vi "SHIFTER - GUI Template.vi"() -> (8 "SHIFTER DATA":T1)   [LabVIEW 2012, in "REx_Springboard.lvlib"]
uses:
  REx_Springboard.lvlib
  TypeDef - SHIFTER - GUI Template.ctl
  Dependencies.llb/Exit Event Ref.ctl
  Dependencies.llb/TLB_Dependencies.lvlib
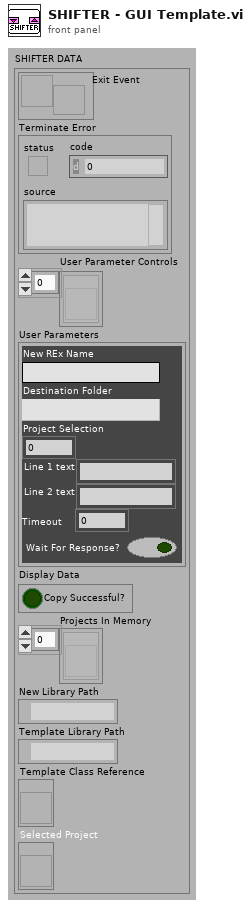
[diagram p1: front panel]
types:
  T1 = typedef "REx_Springboard.lvlib/TypeDef - SHIFTER - GUI Template.ctl" = cluster{"Exit Event":T2, "Terminate Error":errorcluster, "User Parameter Controls":refnum<vi>[], "User Parameters":cluster{"New REx Name":string, "Destination Folder":path, "Project Selection":u16, "Line 1 text":string, "Line 2 text":string, "Timeout":i32, "Wait For Response?":bool}, "Display Data":cluster{"Copy Successful?":bool}, "Projects In Memory":refnum<vi>[], "New Library Path":path, "Template Library Path":path, "Template Class Reference":refnum<vi>, "Selected Project":refnum<vi>}
  T2 = typedef "REx_Springboard.lvlib/TLB_Dependencies.lvlib/Exit Event Ref.ctl" = refnum<user-event>
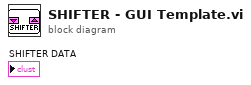
[diagram p0: block diagram]
diagram:
